vi "CalculosParametros.vi"(0 "2D Array":dbl[][](array[numeric]), 1 "Frecuencia \nMuestreo":dbl=5000.0 format="%#_13g") -> (2 "output cluster":T2, 3 "Voltaje":T1, 4 "Corriente":T1)   [LabVIEW 2014]
uses:
  <vilib>/Analysis/5stat.llb/RMS (DBL).vi
  <vilib>/Analysis/baseanly.llb/Mean (DBL).vi
  <vilib>/measure/mascope.llb/Amplitude and Levels 1 chan.vi
  <vilib>/measure/matone.llb/Harmonic Distortion Analyzer 1 Chan.vi
  <vilib>/Analysis/NI_AALBase.lvlib
  <vilib>/measure/NI_MAPro.lvlib
  <vilib>/Analysis/NI_AALPro.lvlib
panel:
  in  "Ajuste de ganancia I":dbl=1.0 format="%#_13g"
  in  "Ajuste de ganancia V":dbl=102.28846559570813 format="%#_13g"
  out "Ip-":dbl format="%.4g"
  out "Ip+":dbl format="%.4g"
  out "Corriete pp":dbl format="%.4p"
  out "Vp-":dbl format="%.4g"
  out "Vp+":dbl format="%.4g"
  out "Voltaje pp":dbl format="%.6p"
  out "Desfasaje prom":dbl
  out "THD I":dbl format="%.2p"
  out "THD V":dbl format="%.2p"
  out "Potencia Reactiva":dbl
  out "FDP":dbl
  out "Potencia Aparente":dbl format="%0.2f"
  out "Frecuencia":dbl format="%.2p"
  out "Potencia \nActiva":dbl format="%0.2f"
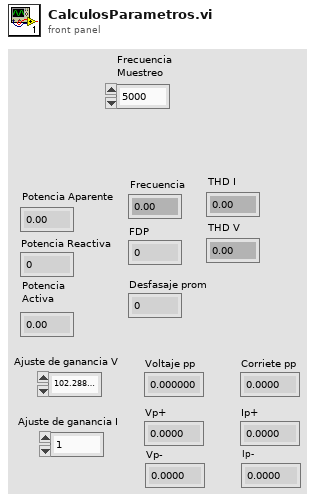
[diagram p1: front panel]
types:
  T1 = cluster{"components level":dbl[], "exported spectrum (dB)":cluster{"f0":dbl, "df":dbl, "dB Spectrum (Hann)":dbl[]}, "Waveform":waveform(dbl), "Power Spectrum (V^2 rms)":dbl[]}
  T2 = cluster{"Frecuencia":dbl, "THD V":dbl, "THD I":dbl, "FDP":dbl, "Potencia Activa":dbl, "Potencia Reactiva":dbl, "Potencia Aparente":dbl, "Desfasaje (FDP)":dbl, "Desfasaje (TM)":dbl, "Flujo":dbl, "Vrms":dbl, "Irms":dbl, "Energia":dbl}
  T3 = enum16{"none", "input signal", "fundamental signal", "residual signal", "harmonics only", "noise and spurs"}
  T4 = cluster{"exported time signal":waveform(dbl), "exported spectrum (dB)":cluster{"f0":dbl, "df":dbl, "dB Spectrum (Hann)":dbl[]}}
  T5 = cluster{"f0":dbl, "df":dbl, "dB Spectrum (Hann)":dbl[]}
  T6 = cluster{"components level":dbl[], "exported spectrum (dB)":cluster{"f0":dbl, "df":dbl, "dB Spectrum (Hann)":dbl[]}, waveform(dbl), "components level":dbl[]}
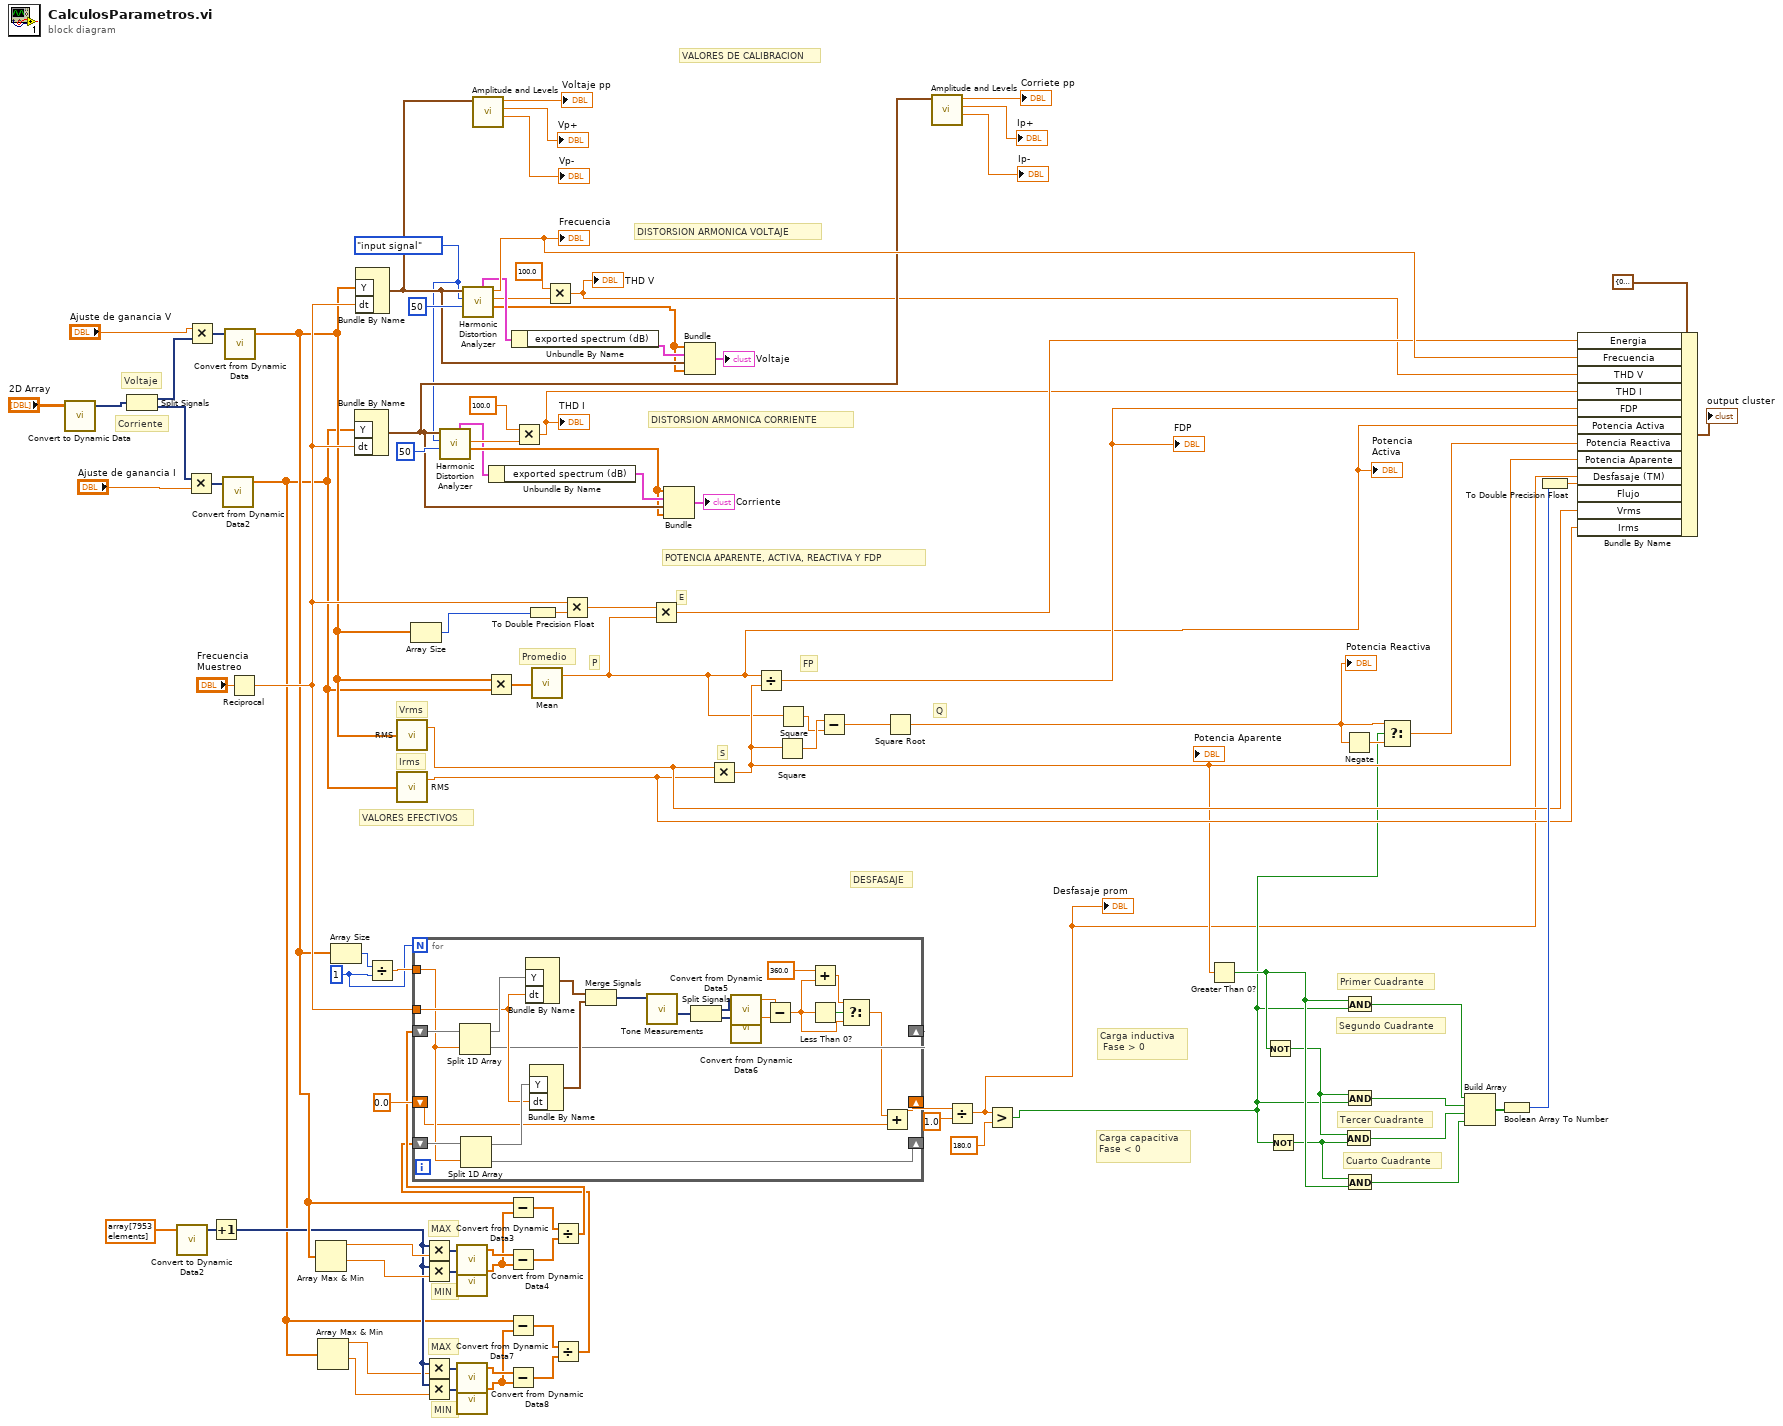
[diagram p0: block diagram]
diagram:
  w37 = T3."input signal" ("export mode")
  w68 = 1
  # "MIN"
  # "MAX"
  # "MIN"
  # "MAX"
  # "FP"
  # "VALORES EFECTIVOS"
  # "VALORES DE CALIBRACION"
  # "S"
  # "E"
  # "Q"
  # "P"
  # "Carga capacitiva \nFase < 0"
  # "Carga inductiva \n Fase > 0"
  # "Cuarto Cuadrante"
  # "Tercer Cuadrante"
  # "Segundo Cuadrante"
  # "Primer Cuadrante"
  # "DISTORSION ARMONICA VOLTAJE"
  # "DISTORSION ARMONICA CORRIENTE"
  # "Promedio"
  # "POTENCIA APARENTE, ACTIVA, REACTIVA Y FDP"
  # "Vrms"
  # "Irms"
  # "DESFASAJE"
  # "Corriente"
  # "Voltaje"
  n1 = call "Convert to Dynamic Data"("2D Array"="2D Array") -> ("Dynamic Data Type"=w76:dynamicdata)  [unwired: 3 in]
  n2 = Split Signals(w76) -> (w75:dynamicdata, w67:dynamicdata)  [unwired: 2 in]
  n3 = call "Convert to Dynamic Data2"("Array"=dbl[] array[7953 elements]) -> ("Dynamic Data Type"=w21:dynamicdata)  [unwired: 3 in]
  n4 = Multiply(x=w67, y="Ajuste de ganancia I") -> (x*y=w66:dynamicdata)
  n5 = Multiply(x="Ajuste de ganancia V", y=w75) -> (x*y=w74:dynamicdata)
  n6 = Increment(x=w21) -> (x+1=w5:dynamicdata)
  n7 = call "Convert from Dynamic Data2"("Dynamic Data Type"=w66) -> ("Array"=w4:dbl[])  [unwired: 3 in]
  n8 = call "Convert from Dynamic Data"("Dynamic Data Type"=w74) -> ("Array"=w23:dbl[])  [unwired: 3 in]
  n9 = Reciprocal(x="Frecuencia \nMuestreo") -> (1/x=w43:dbl)
  n10 = Array Max & Min(array=w23) -> (max value=w20:dbl, min value=w6:dbl)  [unwired: 2 out]
  n11 = Array Max & Min(array=w4) -> (max value=w3:dbl, min value=w7:dbl)  [unwired: 2 out]
  n12 = Array Size(array=w23) -> (size(s)=w69:i32)
  n13 = Bundle By Name("Y"=w4, "dt"=w43) -> (w44:waveform(dbl))  [unwired: 1 in]
  n14 = Bundle By Name("Y"=w23, "dt"=w43) -> (w51:waveform(dbl))  [unwired: 1 in]
  n15 = Divide(x=w69, y=w68) -> (x/y=w70:dbl)
  n16 = call-poly <vilib>:"RMS.vi"("X"=w23) -> ("rms value"=w83:dbl)  [unwired: 1 out]
  n17 = call-poly <vilib>:"RMS.vi"("X"=w4) -> ("rms value"=w82:dbl)  [unwired: 1 out]
  n18 = Array Size(array=w23) -> (size(s)=w60:i32)
  n19 = Multiply(x=w5, y=w20) -> (x*y=w19:dynamicdata)
  n20 = Multiply(x=w5, y=w6) -> (x*y=w18:dynamicdata)
  n21 = Multiply(x=w5, y=w3) -> (x*y=w13:dynamicdata)
  n22 = Multiply(x=w5, y=w7) -> (x*y=w12:dynamicdata)
  n23 = call-poly <vilib>:"Harmonic Distortion Analyzer.vi"("highest harmonic"=50, "export mode"=w37, "signal in"=w44) -> ("components level"=w25:dbl[], "THD"=w35:dbl, "exported signals"=w24:T4)  [unwired: 3 in, 3 out]
  n24 = call "Convert from Dynamic Data3"("Dynamic Data Type"=w19) -> ("Array"=w17:dbl[])  [unwired: 3 in]
  n25 = call "Convert from Dynamic Data4"("Dynamic Data Type"=w18) -> ("Array"=w16:dbl[])  [unwired: 3 in]
  n26 = call "Convert from Dynamic Data7"("Dynamic Data Type"=w13) -> ("Array"=w11:dbl[])  [unwired: 3 in]
  n27 = call "Convert from Dynamic Data8"("Dynamic Data Type"=w12) -> ("Array"=w10:dbl[])  [unwired: 3 in]
  n28 = call-poly <vilib>:"Harmonic Distortion Analyzer.vi"("highest harmonic"=50, "export mode"=w37, "signal in"=w51) -> ("components level"=w26:dbl[], "THD"=w32:dbl, "detected fundamental frequency"=w94:dbl, "exported signals"=w39:T4)  [unwired: 3 in, 2 out]
  "Frecuencia" <- w94
  n29 = call-poly <vilib>:"Amplitude and Levels.vi"("signal in"=w51) -> ("low state level"=→"Vp-":dbl, "high state level"=→"Vp+":dbl, "amplitude"=→"Voltaje pp":dbl)  [unwired: 7 in, 1 out]
  n30 = Multiply(x=w23, y=w4) -> (x*y=w96:dbl[])
  n31 = Unbundle By Name(w24) -> ("exported spectrum (dB)"=w41:T5)
  n32 = Subtract(x=w23, y=w16) -> (x-y=w15:dbl[])
  n33 = Subtract(x=w17, y=w16) -> (x-y=w14:dbl[])
  n34 = Subtract(x=w4, y=w10) -> (x-y=w9:dbl[])
  n35 = Subtract(x=w11, y=w10) -> (x-y=w8:dbl[])
  n36 = Unbundle By Name(w39) -> ("exported spectrum (dB)"=w38:T5)
  n37 = Multiply(x=100.0, y=w35) -> (x*y=w36:dbl)
  "THD I" <- w36
  n38 = To Double Precision Float(number=w60) -> (double precision float=w61:dbl)
  n39 = call-poly <vilib>:"Mean.vi"("X"=w96) -> ("mean"=w56:dbl)  [unwired: 1 out]
  "Potencia \nActiva" <- w56
  n40 = Multiply(x=100.0, y=w32) -> (x*y=w33:dbl)
  "THD V" <- w33
  n41 = Divide(x=w15, y=w14) -> (x/y=w2:dbl[])
  n42 = Divide(x=w9, y=w8) -> (x/y=w1:dbl[])
  n43 = for {
    N: w68 -> [_]
    shift-right: [w106] -> _
    shift-left: w2 -> [w119]
    tunnel: w43 -> [w115]
    shift-right: [w102] -> _
    shift-left: w1 -> [w116]
    shift-right: [w108] -> w30
    shift-left: 0.0 -> [w103]
    tunnel: w70 -> [w104]
    n44 = Split 1D Array(array=w119, index=w104) -> (first subarray=w118:dbl[], second subarray=w106:dbl[])
    n45 = Split 1D Array(array=w116, index=w104) -> (first subarray=w117:dbl[], second subarray=w102:dbl[])
    n46 = Bundle By Name ("Build Waveform")("Y"=w118, "dt"=w115) -> (w105:waveform(dbl))  [unwired: 1 in]
    n47 = Bundle By Name("Y"=w117, "dt"=w115) -> (w114:waveform(dbl))  [unwired: 1 in]
    n48 = Merge Signals(w105, w114) -> (w107:dynamicdata)
    n49 = call "Tone Measurements"("Signals"=w107) -> ("Phase"=w110:dynamicdata)  [unwired: 9 in, 1 out]
    n50 = Split Signals(w110) -> (w109:dynamicdata, w113:dynamicdata)  [unwired: 2 in]
    n51 = call "Convert from Dynamic Data5"("Dynamic Data Type"=w109) -> ("Scalar"=w112:dbl)  [unwired: 3 in]
    n52 = call "Convert from Dynamic Data6"("Dynamic Data Type"=w113) -> ("Scalar"=w111:dbl)  [unwired: 3 in]
    n53 = Subtract(x=w112, y=w111) -> (x-y=w97:dbl)
    n54 = Add(x=360.0 ("y"), y=w97) -> (x+y=w99:dbl)
    n55 = Less Than 0?(x=w97) -> (x < 0?=w101:bool)
    n56 = Select(t=w99, s=w101, f=w97) -> (s? t:f=w100:dbl)
    n57 = Add(x=w100, y=w103) -> (x+y=w108:dbl)
  }
  n58 = Multiply(x=w43, y=w61) -> (x*y=w62:dbl)
  n59 = Multiply(x=w62, y=w56) -> (x*y=w58:dbl)
  n60 = Bundle("components level"=w25, "exported spectrum (dB)"=w41, w44, "components level"=w25) -> (→"Corriente":T6)  [unwired: 1 in]
  n61 = Bundle("components level"=w26, "exported spectrum (dB)"=w38, w51, "components level"=w26) -> (→"Voltaje":T6)  [unwired: 1 in]
  n62 = Multiply(x=w83, y=w82) -> (x*y=w57:dbl)
  "Potencia Aparente" <- w57
  n63 = Divide(x=w56, y=w57) -> (x/y=w85:dbl)
  "FDP" <- w85
  n64 = Square(x=w57) -> (x^2=w55:dbl)
  n65 = Square(x=w56) -> (x^2=w54:dbl)
  n66 = Subtract(x=w55, y=w54) -> (x-y=w53:dbl)
  n67 = Square Root(x=w53) -> (sqrt(x)=w52:dbl)
  "Potencia Reactiva" <- w52
  n68 = call-poly <vilib>:"Amplitude and Levels.vi"("signal in"=w44) -> ("low state level"=→"Ip-":dbl, "high state level"=→"Ip+":dbl, "amplitude"=→"Corriete pp":dbl)  [unwired: 7 in, 1 out]
  n69 = Divide(x=w30, y=1.0) -> (x/y=w27:dbl)
  "Desfasaje prom" <- w27
  n70 = Greater?(x=w27, y=180.0) -> (0:w28:bool)
  n71 = Greater Than 0?(x=w57) -> (x > 0?=w86:bool)
  n72 = Not(x=w86) -> (.not. x?=w81:bool)
  n73 = Not(x=w28) -> (.not. x?=w80:bool)
  n74 = Negate(x=w52) -> (-x=w78:dbl)
  n75 = And(x=w81, y=w80) -> (x .and. y?=w90:bool)
  n76 = And(x=w86, y=w28) -> (x .and. y?=w92:bool)
  n77 = And(x=w81, y=w28) -> (x .and. y?=w91:bool)
  n78 = And(x=w80, y=w86) -> (x .and. y?=w89:bool)
  n79 = Select(t=w52, s=w28, f=w78) -> (s? t:f=w79:dbl)
  n80 = Build Array(w92, w91, w90, w89) -> (w88:bool[])
  n81 = Boolean Array To Number(Boolean array=w88) -> (number=w87:u32)
  n82 = To Double Precision Float(number=w87) -> (double precision float=w84:dbl)
  n83 = Bundle By Name(cluster=T2 {"Frecuencia"=0.0, "THD V"=0.0, "THD I"=0.0, "FDP"=0.0, "Potencia Activa"=0.0, "Potencia Reactiva"=0.0, "Potencia Aparente"=0.0, "Desfasaje (FDP)"=0.0, "Desfasaje (TM)"=0.0, "Flujo"=0.0, "Vrms"=0.0, "Irms"=0.0, "Energia"=0.0}, "Energia"=w58, "Frecuencia"=w94, "THD V"=w33, "THD I"=w36, "FDP"=w85, "Potencia Activa"=w56, "Potencia Reactiva"=w79, "Potencia Aparente"=w57, "Desfasaje (TM)"=w27, "Flujo"=w84, "Vrms"=w83, "Irms"=w82) -> (→"output cluster":T2)
